vi "PID.vi"(3 "dt(s)":dbl=-1.0 format="%.3f", 4 "s":dbl=-1.0 format="%.3f", 6 "error in (no error)":errorcluster, 7 "Reset":bool, 9 "Enum":enum16{"M4", "M3", "M2", "M1"}(ring)) -> (0 "error out 2":errorcluster, 2 "en/deg":dbl)   [LabVIEW 2018]
uses:
  <vilib>/addons/control/pid/pid.llb/PID (DBL).vi
  <vilib>/addons/control/pid/NI_PID_pid.lvlib
panel:
  out "Waveform Chart":cluster{"s":dbl, "en/deg":dbl}(graph)
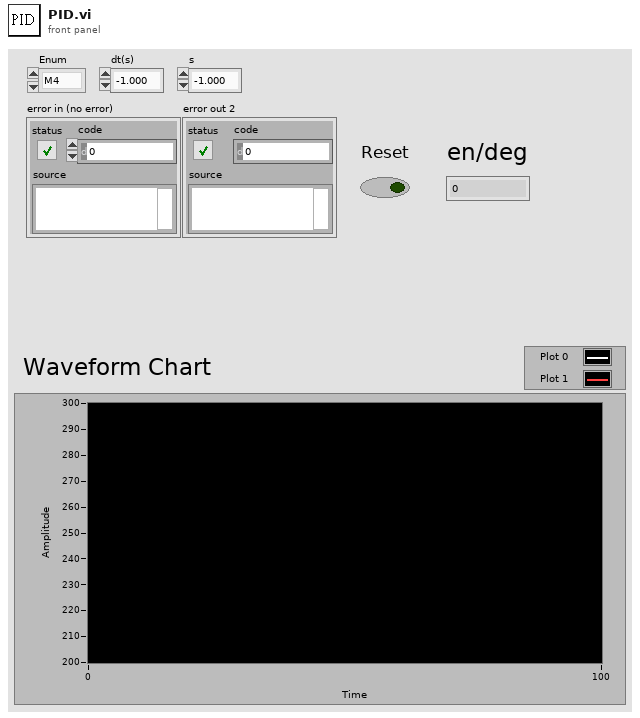
[diagram p1: front panel]
types:
  T1 = cluster{"proportional gain (Kc)":dbl, "integral time (Ti, min)":dbl, "derivative time (Td, min)":dbl}
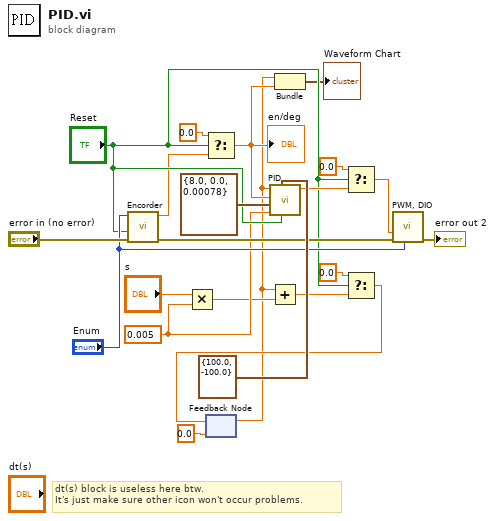
[diagram p0: block diagram]
diagram:
  w7 = 0.005 ("dt (s)")
  # "dt(s) block is useless here btw.\nIt's just make sure other icon won't occur problems."
  n1 = call "Encorder.vi"("error in (no error)"="error in (no error)", "Reset Counter"="Reset", "Enum"="Enum") -> ("error out"=w17:errorcluster, "en/deg"=w9:dbl)  [unwired: 6 in]
  n2 = Multiply(x="s", y=w7) -> (x*y=w6:dbl)
  n3 = Select(t=0.0, s="Reset", f=w9) -> (s? t:f=w8:dbl)
  "en/deg" <- w8
  n4 = feedback #1(0.0 ("t")) -> (w1:dbl)
  n5 = call-poly <vilib>:"PID.vi"("reinitialize? (F)"="Reset", "output range"=cluster{"output high":dbl, "output low":dbl} {"output high"=100.0, "output low"=-100.0}, "dt (s)"=w7, "PID gains"=T1 {"proportional gain (Kc)"=8.0, "integral time (Ti, min)"=0.0, "derivative time (Td, min)"=0.00078}, "process variable"=w8, "setpoint"=w1) -> ("output"=w14:dbl)  [unwired: 4 in, 1 out]
  n6 = Add(x=w1, y=w6) -> (x+y=w5:dbl)
  n7 = Bundle("t"=w1, "en/deg"=w8) -> (→"Waveform Chart":cluster{"t":dbl, "en/deg":dbl})  [unwired: 1 in]
  n8 = Select(t=0.0, s="Reset", f=w14) -> (s? t:f=w11:dbl)
  n9 = Select(t=0.0, s="Reset", f=w5) -> (s? t:f=w4:dbl)
  n10 = feedback-in #1(w4) -> ()
  n11 = call "PWM, DIO.vi"("Enum"="Enum", "error in (no error)"=w17, "PWM"=w11) -> ("error out 2"=→"error out 2":errorcluster)  [unwired: 8 in]
